vi "Send Shutdown.vi"(8 "error in (no error)":errorcluster, 11 "Logging Interface in":refnum<class "Logging Interface.lvclass">) -> (0 "error out":errorcluster, 3 "Logging Interface out":refnum<class "Logging Interface.lvclass">)   [LabVIEW 2020, in "DSF Core.lvlib" / "Logging Interface.lvclass"]
uses:
  Logging Interface.lvclass
  Interface.lvclass
  Send Logging Command.vi
  Command.ctl
  Parameters.ctl
  Command Data.ctl
  Wait For Logging Response.vi
  Response.ctl
  Dispatcher/Invalid Response.vi
  C:/Users/nitest/Desktop/Git/niveristand-data-sharing-framework-custom-device/Source/Core/Classes/Interface/Interface.lvclass
  C:/Users/nitest/Desktop/Git/niveristand-data-sharing-framework-custom-device/Source/Core/Classes/Interface/Logging/Logging Interface.lvclass
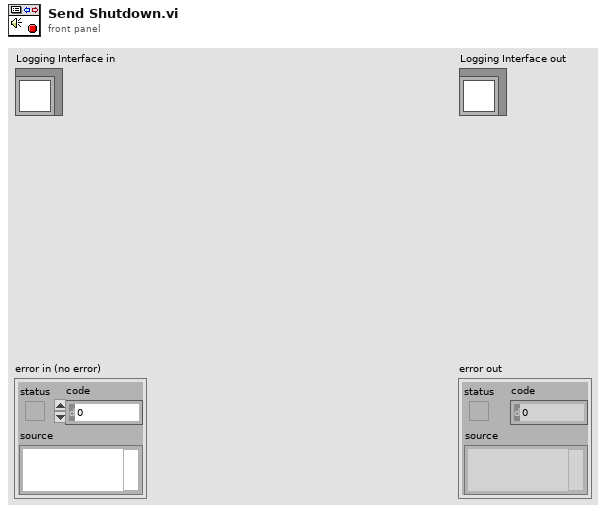
[diagram p1: front panel]
types:
  T1 = typedef "DSF Core.lvlib/Logging Interface.lvclass/Command.ctl" = enum8{"Idle", "Start", "Log Framework State", "Log Plugin State", "Log Dispatcher State", "Shutdown"}
  T2 = typedef "DSF Core.lvlib/Logging Interface.lvclass/Command Data.ctl" = cluster{"Command":T1, "Parameters":T3}
  T3 = typedef "DSF Core.lvlib/Logging Interface.lvclass/Parameters.ctl" = cluster{"arg1":u64, "arg2":u64}
  T4 = typedef "DSF Core.lvlib/Logging Interface.lvclass/Response Data.ctl" = cluster{"Response":T5, "Parameters":T3}
  T5 = typedef "DSF Core.lvlib/Logging Interface.lvclass/Response.ctl" = enum8{"General Ack", "Error", "Shutting Down"}
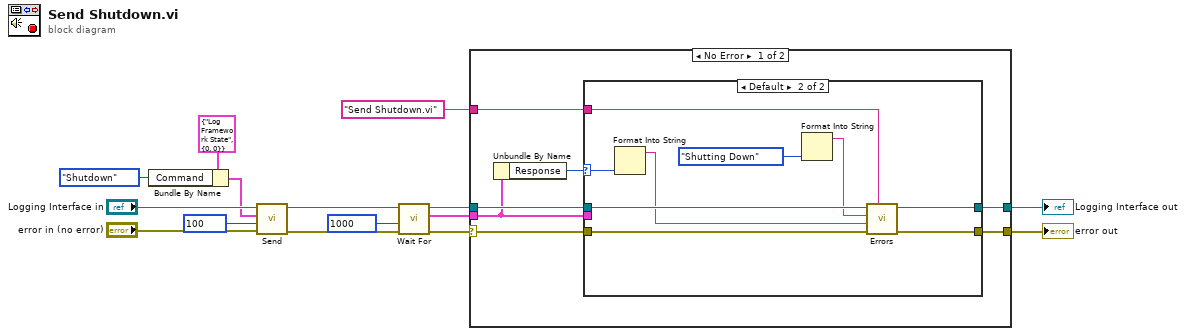
[diagram p0: block diagram]
diagram:
  n1 = Bundle By Name(cluster=T2 {"Command"=enum."Log Framework State", "Parameters"={"arg1"=0, "arg2"=0}} ("command"), "Command"=Command."Shutdown") -> (w12:T2)
  n2 = call-poly "Send.vi"("error in (no error)"="error in (no error)", "timeout in ms (0)"=100, "command"=w12, "Logging Interface in"="Logging Interface in") -> ("error out"=w5:errorcluster, "Logging Interface out"=w4:refnum<class "Logging Interface.lvclass">)  [unwired: 6 in]
  n3 = call-poly "Wait For.vi"("error in (no error)"=w5, "timeout in ms (0)"=1000, "Logging Interface in"=w4) -> ("error out"=w7:errorcluster, "response"=w8:T4, "Logging Interface out"=w10:refnum<class "Logging Interface.lvclass">)  [unwired: 5 in, 1 out]
  n4 = case shown="No Error" w7 {
    selector: w7 -> [w17 w34]
    tunnel: [w21 w34] -> w3
    tunnel: w10 -> [w20 w35]
    tunnel: [w19 w35] -> w2
    tunnel: w8 -> [w18 _]
    tunnel: "Send Shutdown.vi" ("error source vi name") -> [w16 _]
    frame No Error {
      n5 = Unbundle By Name(w18) -> ("Response"=w22:T5)
      n6 = case shown="Default" w22 {
        selector: w22 -> [_ w28]
        tunnel: w17 -> [w23 w32]
        tunnel: [w23 w30] -> w21
        tunnel: w20 -> [w24 w33]
        tunnel: [w24 w31] -> w19
        tunnel: w18 -> [_ _]
        tunnel: w16 -> [_ w29]
        frame "Shutting Down" {
        }
        frame Default {
          n7 = Format Into String(w28) -> (resulting string=w27:string)  [unwired: 3 in, 1 out]
          n8 = Format Into String(Response."Shutting Down" ("expected response")) -> (resulting string=w25:string)  [unwired: 3 in, 1 out]
          n9 = call-poly "Errors.vi"("error source vi name"=w29, "error in (no error)"=w32, "actual response"=w27, "expected response"=w25, "Interface in"=w33) -> ("error out"=w30:errorcluster, "Interface out"=w31:refnum<class "Logging Interface.lvclass">)  [unwired: 5 in]
        }
      }
    }
    frame Error {
      # "Incoming error. Pass through."
    }
  }
  "error out" <- w3
  "Logging Interface out" <- w2
